vi "ParseAnemoString.vi"(11 "String":string) -> (0 "SupplyVolts":dbl, 1 "N,E Components":dbl[](array[numeric]) format="%.4f", 2 "direction":dbl, 3 "speed":dbl, 4 "999Error":dbl, 6 "ParseError":dbl)   [LabVIEW 2015]
panel:
  out "SerialNo":i32
  out "SerialAlpha":string
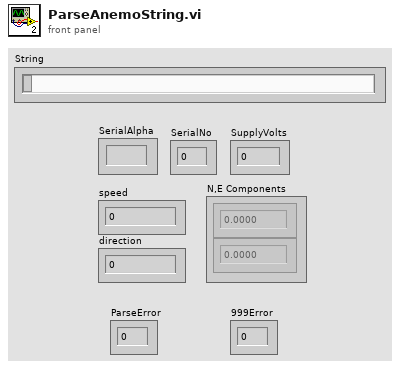
[diagram p1: front panel]
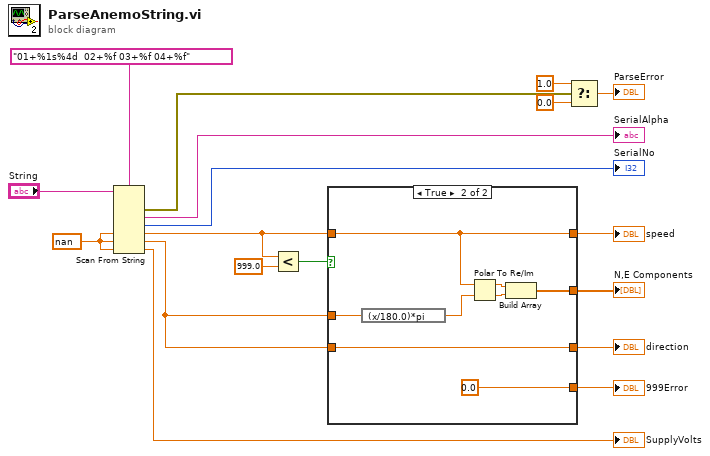
[diagram p0: block diagram]
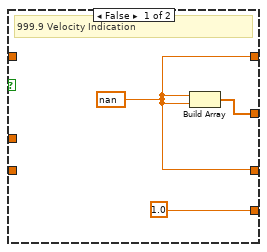
[diagram p2: hidden frame]
diagram:
  w6 = nan ("default value 2")
  n1 = Scan From String(format string="01+%1s%4d  02+%f 03+%f 04+%f", input string="String", default 3=w6, default 4=w6, default 5=w6) -> (error out=w5:errorcluster, output 1=→"SerialAlpha":string, output 2=→"SerialNo":i32, output 3=w8:dbl, output 4=w9:dbl, output 5=→"SupplyVolts":dbl)  [unwired: 4 in, 2 out]
  n2 = Less?(x=w8, y=999.0) -> (x < y?=w14:bool)
  n3 = case shown="True" w14 {
    tunnel: w9 -> [_ w28]
    tunnel: [w21 w25] -> w16
    tunnel: w8 -> [_ w24]
    tunnel: [w20 w24] -> w13
    tunnel: w9 -> [_ w23]
    tunnel: [w20 w23] -> w12
    tunnel: [1.0 0.0 ("999Error")] -> w1
    frame False {
      w20 = nan
      # "999.9 Velocity Indication"
      n4 = Build Array(w20, w20) -> (w21:dbl[])
    }
    frame True {
      n5 = expression code="(x/180.0)*pi" ("degrees to radians")(w28) -> (w29:dbl)
      n6 = Polar To Re/Im(2:w29, 3:w24) -> (0:w26:dbl, 1:w27:dbl)
      n7 = Build Array(w27, w26) -> (w25:dbl[])
    }
  }
  "speed" <- w13
  "direction" <- w12
  "N,E Components" <- w16
  "999Error" <- w1
  n8 = Select(t=1.0, s=w5, f=0.0) -> (s? t:f=→"ParseError":dbl)
